vi "Query Slew Rate (All).vi"(0 "VISA resource name":refnum<visa-resource-name>, 11 "error in (no error)":errorcluster) -> (4 "VISA resource name out":refnum<visa-resource-name>, 6 "Voltage Slew Rate (V per sec)":dbl format="%#.6g", 8 "Current Slew Rate (A per sec)":dbl format="%#.6g", 10 "Power Slew Rate (W per sec)":dbl format="%#.6g", 14 "Resistance Slew Rate (Ohms per sec)":dbl format="%#.6g", 15 "error out":errorcluster)   [LabVIEW 2020, in "NH Research Regenerative Test Series.lvlib"]
doc: "Returns the slew rate for all programmed changes in the voltage, current, power, and resistance output of the module. This command returns both positive and negative going slew rates."
uses:
  NH Research Regenerative Test Series.lvlib
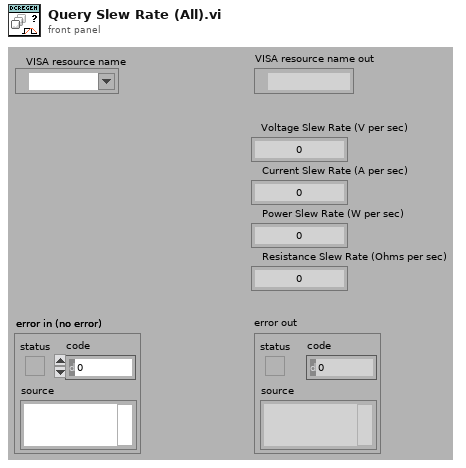
[diagram p1: front panel]
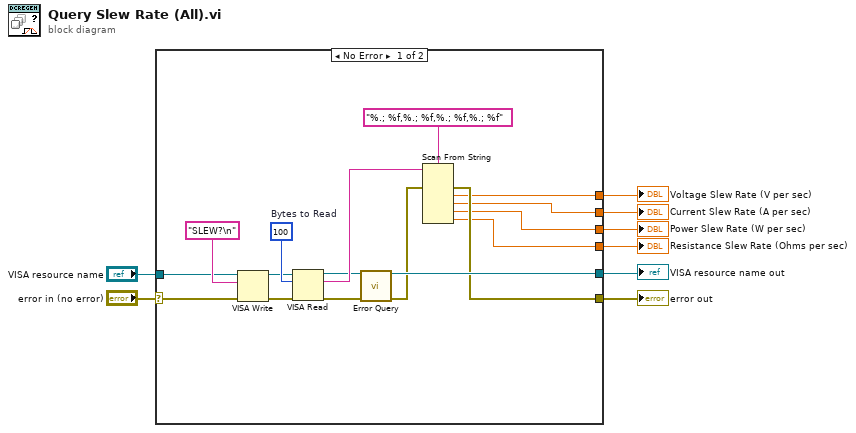
[diagram p0: block diagram]
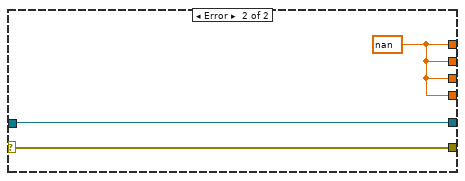
[diagram p2: hidden frame]
diagram:
  n1 = case shown="No Error" "error in (no error)" {
    selector: "error in (no error)" -> [w21 w28]
    tunnel: [w13 w28] -> w7
    tunnel: [w17 w27] -> w5
    tunnel: "VISA resource name" -> [w20 w27]
    tunnel: [w12 w26] -> w4
    tunnel: [w11 w26] -> w3
    tunnel: [w10 w26] -> w2
    tunnel: [w9 w26] -> w1
    frame No Error {
      w25 = u32 100  # Bytes to Read
      n2 = VISA Write(VISA resource name=w20, write buffer="SLEW?\n", error in (no error)=w21) -> (VISA resource name out=w23:refnum<visa-resource-name>, error out=w24:errorcluster)  [unwired: 1 out]
      n3 = VISA Read(VISA resource name=w23, byte count=w25, error in (no error)=w24) -> (VISA resource name out=w16:refnum<visa-resource-name>, read buffer=w19:string, error out=w15:errorcluster)  [unwired: 1 out]
      n4 = call "Error Query.vi"("VISA resource name"=w16, "error in (no error)"=w15) -> ("VISA resource name out"=w17:refnum<visa-resource-name>, "error out"=w14:errorcluster)  [unwired: 10 in, 2 out]
      n5 = Scan From String(format string="%.; %f,%.; %f,%.; %f,%.; %f", input string=w19, error in=w14) -> (error out=w13:errorcluster, output 1=w12:dbl, output 2=w11:dbl, output 3=w10:dbl, output 4=w9:dbl)  [unwired: 5 in, 2 out]
    }
    frame Error {
      w26 = nan
    }
  }
  "error out" <- w7
  "VISA resource name out" <- w5
  "Voltage Slew Rate (V per sec)" <- w4
  "Current Slew Rate (A per sec)" <- w3
  "Power Slew Rate (W per sec)" <- w2
  "Resistance Slew Rate (Ohms per sec)" <- w1
